vi "AI-Motor-Read.vi"(10 "Error In":errorcluster) -> (2 "Error Out":errorcluster, 3 "Data":dbl)   [LabVIEW 2019]
uses:
  <instrlib>/Dynamixel Motor/Public/Motor Operation/Low Level/Baud Setting.ctl
  Variable/Position.vi
  <instrlib>/Dynamixel Motor/Dynamixel Motor.lvlib
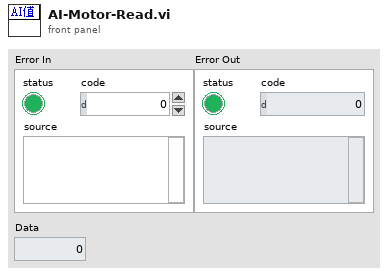
[diagram p1: front panel]
types:
  T1 = typedef "Dynamixel Motor.lvlib/Baud Setting.ctl" = u8
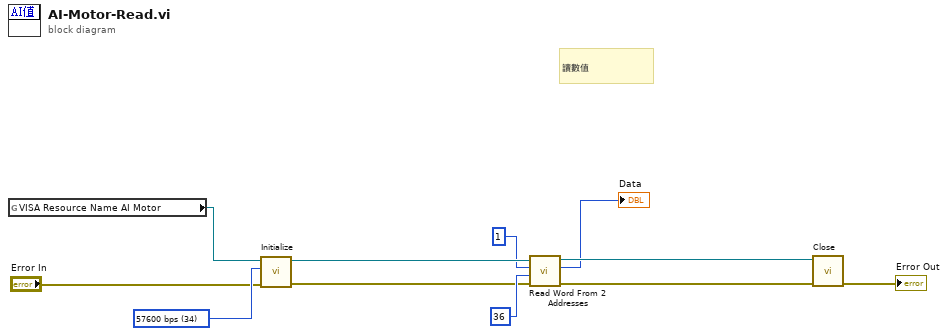
[diagram p0: block diagram]
diagram:
  w11 = T1 34 items=["1,000,000 bps"=1, "500,000 bps"=3, "400,000 bps"=4, "250,000 bps"=7, "200,000 bps"=9, "115200 bps"=16, "57600 bps"=34, "19200 bps"=103, "9600 bps"=207] ("Baud rate (57600 bps)")
  # "讀數值"
  n1 = global read "Position.vi" "VISA Resource Name AI Motor"() -> (w1:refnum<visa-resource-name>)
  n2 = call <instrlib>:"Initialize.vi"("error in (no error)"="Error In", "Baud rate (57600 bps)"=w11, "VISA resource name"=w1) -> ("error out"=w4:errorcluster, "VISA resource name out"=w5:refnum<visa-resource-name>)  [unwired: 7 in]
  n3 = call <instrlib>:"Read Word From 2 Addresses.vi"("Error in (no error)"=w4, "Address number (0)"=u8 36, "Motor ID (0)"=u8 1, "VISA resource name"=w5) -> ("error out"=w10:errorcluster, "Data"=→"Data":u16, "VISA resource name out"=w9:refnum<visa-resource-name>)  [unwired: 5 in]
  n4 = call <instrlib>:"Close.vi"("error in (no error)"=w10, "VISA resource name"=w9) -> ("error out"=→"Error Out":errorcluster)  [unwired: 9 in]
